vi "configREF_phi.vi"(7 "address":string, 8 "error in (no error)":errorcluster, 9 "new phi (deg)":dbl, 10 "lockin Channel":i32, 11 "Channels: Lockin":T1={"REF f (Hz)"=[13.0], "REF phi (deg)"=[0.0]} {"REF phi (deg)" format="%#_3g"}) -> (0 "error out":errorcluster, 3 "Channels: Lockin":T1={"REF f (Hz)"=[13.0], "REF phi (deg)"=[0.0]} {"REF phi (deg)" format="%#_3g"})   [LabVIEW 2016]
doc: "API to configure a REF phase.\n\nSpecify which channel you want to change and the value you want to set.\n\nIf address=\"\", this API reads from localhost\nIf address is remote lockin, you need to add this computer to allowed whitelist on the lockin computer you are trying to access."
uses:
  Typedefs/REF-cluster.ctl
  Typedefs/REF_f-array.ctl
  Typedefs/REF_phi-array.ctl
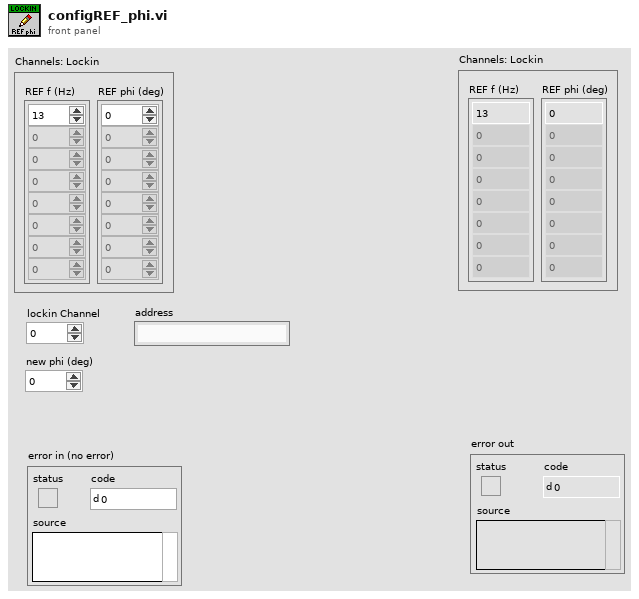
[diagram p1: front panel]
types:
  T1 = typedef "REF-cluster.ctl" = cluster{"REF f (Hz)":T2, "REF phi (deg)":T3}
  T2 = typedef "REF_f-array.ctl" = dbl[]
  T3 = typedef "REF_phi-array.ctl" = dbl[]
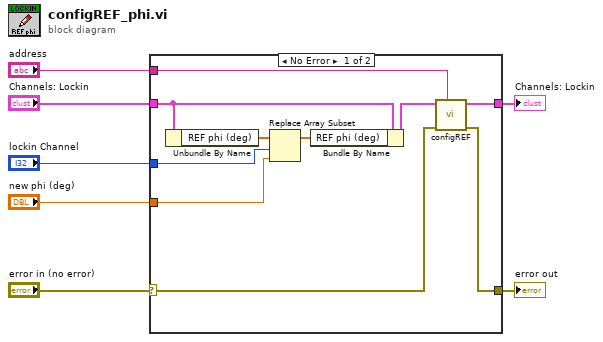
[diagram p0: block diagram]
diagram:
  n1 = case shown="No Error" "error in (no error)" {
    selector: "error in (no error)" -> [w10 w19]
    tunnel: "Channels: Lockin" -> [w15 w18]
    tunnel: [w11 w18] -> w6
    tunnel: "lockin Channel" -> [w14 _]
    tunnel: "new phi (deg)" -> [w13 _]
    tunnel: [w9 w19] -> w2
    tunnel: "address" -> [w8 _]
    frame No Error {
      n2 = Unbundle By Name(w15) -> ("REF phi (deg)"=w16:T3)
      n3 = Replace Array Subset(array=w16, new element=w13, index=w14) -> (w17:T3)
      n4 = Bundle By Name(cluster=w15, "REF phi (deg)"=w17) -> (w12:T1)
      n5 = call "configREF.vi"("address"=w8, "error in (no error)"=w10, "Channels: Lockin in"=w12) -> ("error out"=w9:errorcluster, "Channels: Lockin out"=w11:T1)  [unwired: 7 in]
    }
    frame Error {
    }
  }
  "Channels: Lockin" <- w6
  "error out" <- w2
